vi "KH7008 Control Panel.vi"() -> ()   [LabVIEW 2013]
uses:
  <vilib>/Utility/xml.llb/Write to XML File(string).vi
  <vilib>/Utility/xml.llb/Read From XML File(string).vi
panel:
  in  "Device Number":i32=113885
  in  "Old Settings":T1(array[cluster])=[{"Gain"=1, "Input Coupling"=3, "Shunt Resistor"=1, "Coupling"=1, "Bandwidth Filter"=2}, {"Gain"=1, "Input Coupling"=3, "Shunt Resistor"=1, "Coupling"=1, "Bandwidth Filter"=2}, {"Gain"=1, "Input Coupling"=3, "Shunt Resistor"=1, "Coupling"=1, "Bandwidth Filter"=2}, {"Gain"=1, "Input Coupling"=3, "Shunt Resistor"=1, "Coupling"=1, "Bandwidth Filter"=2}, {"Gain"=1, "Input Coupling"=3, "Shunt Resistor"=1, "Coupling"=1, "Bandwidth Filter"=2}, {"Gain"=1, "Input Coupling"=3, "Shunt Resistor"=1, "Coupling"=1, "Bandwidth Filter"=2}, {"Gain"=1, "Input Coupling"=3, "Shunt Resistor"=1, "Coupling"=1, "Bandwidth Filter"=2}, {"Gain"=1, "Input Coupling"=3, "Shunt Resistor"=1, "Coupling"=1, "Bandwidth Filter"=2}] {"Bandwidth Filter" items=["OFF"=1, "ON"=2]; "Coupling" items=["AC"=1, "DC"=2]; "Shunt Resistor" items=["Open"=1, "50"=2, "500"=3, "5k"=4, "50k"=5]; "Input Coupling" items=["Off"=1, "SE +"=2, "SE -"=3, "Diff"=4]; "Gain" items=["1x"=1, "10x"=2, "100x"=3, "1000x"=4]}
  in  "Load":bool
  in  "Save":bool
  in  "File Identifier (for save)":string
  out "Working":bool
  in  "Refresh":bool
  in  "Settings":T1(array[cluster])=[{"Gain"=1, "Input Coupling"=3, "Shunt Resistor"=1, "Coupling"=1, "Bandwidth Filter"=2}, {"Gain"=1, "Input Coupling"=3, "Shunt Resistor"=1, "Coupling"=1, "Bandwidth Filter"=2}, {"Gain"=1, "Input Coupling"=3, "Shunt Resistor"=1, "Coupling"=1, "Bandwidth Filter"=2}, {"Gain"=1, "Input Coupling"=3, "Shunt Resistor"=1, "Coupling"=1, "Bandwidth Filter"=2}, {"Gain"=1, "Input Coupling"=3, "Shunt Resistor"=1, "Coupling"=1, "Bandwidth Filter"=2}, {"Gain"=1, "Input Coupling"=3, "Shunt Resistor"=1, "Coupling"=1, "Bandwidth Filter"=2}, {"Gain"=1, "Input Coupling"=3, "Shunt Resistor"=1, "Coupling"=1, "Bandwidth Filter"=2}, {"Gain"=1, "Input Coupling"=3, "Shunt Resistor"=1, "Coupling"=1, "Bandwidth Filter"=2}] {"Bandwidth Filter" items=["OFF"=1, "ON"=2]; "Coupling" items=["AC"=1, "DC"=2]; "Shunt Resistor" items=["Open"=1, "50"=2, "500"=3, "5k"=4, "50k"=5]; "Input Coupling" items=["Off"=1, "SE +"=2, "SE -"=3, "Diff"=4]; "Gain" items=["1x"=1, "10x"=2, "100x"=3, "1000x"=4]}
  in  "VISA resource name":refnum<visa-resource-name>="COM3"
  # "Input\nCoupling"
  # "Shunt\nResistor"
  # "Bandwidth\nFilter"
  # "Gain"
  # "Coupling"
  # "CH 1"
  # "CH 2"
  # "CH 3"
  # "CH 4"
  # "CH 5"
  # "CH 6"
  # "CH 7"
  # "CH 8"
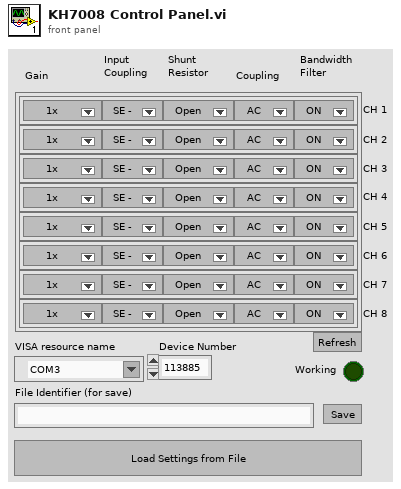
[diagram p1: front panel]
types:
  T1 = cluster{"Gain":u16, "Input Coupling":u16, "Shunt Resistor":u16, "Coupling":u16, "Bandwidth Filter":u16}[]
  T2 = cluster{"Gain":u16, "Input Coupling":u16, "Shunt Resistor":u16, "Coupling":u16, "Bandwidth Filter":u16}
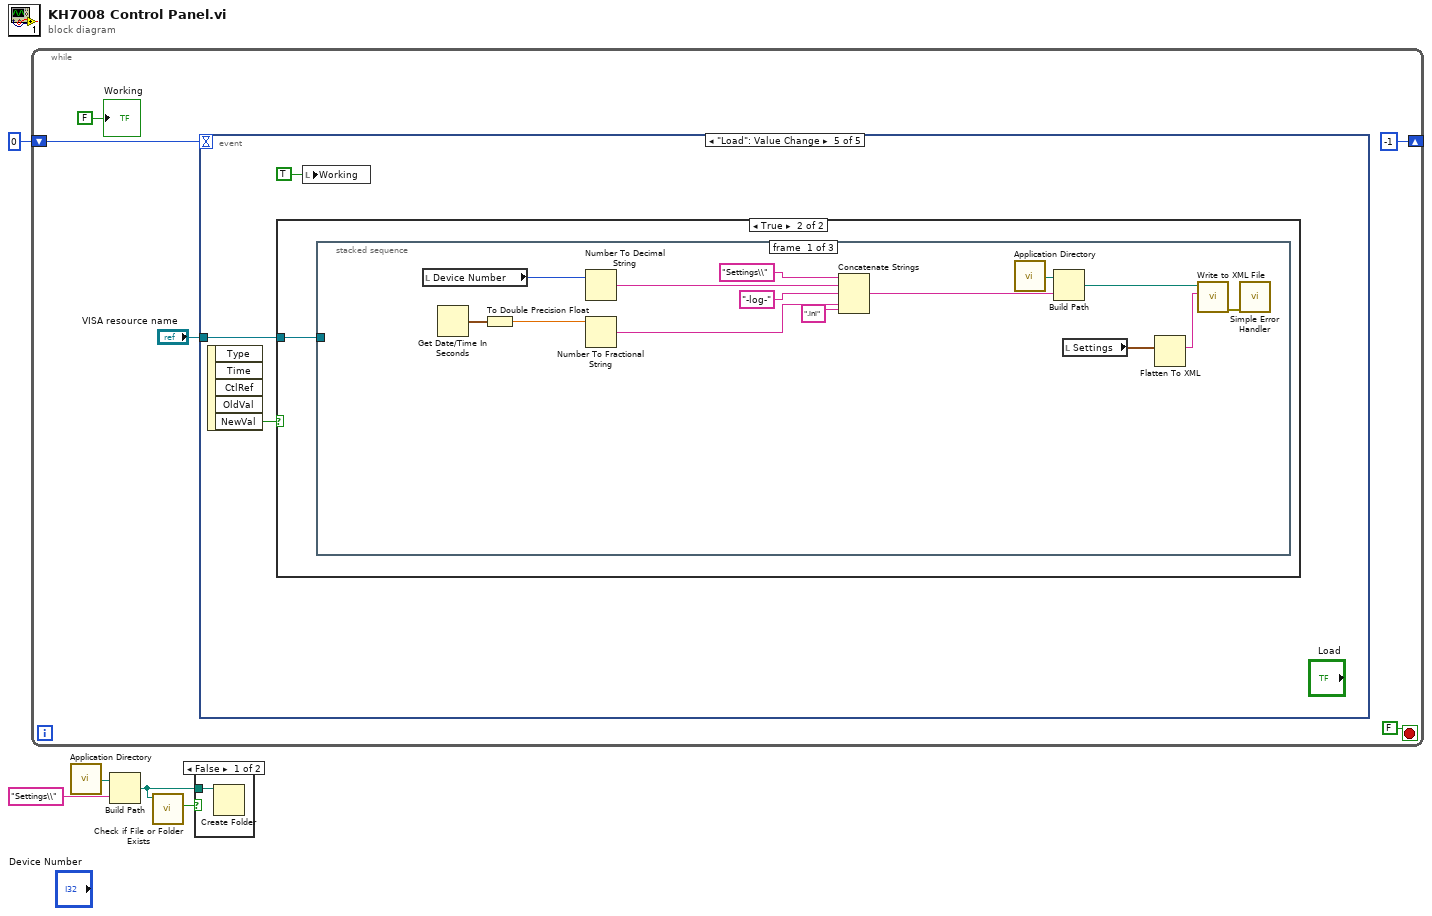
[diagram p0: block diagram]
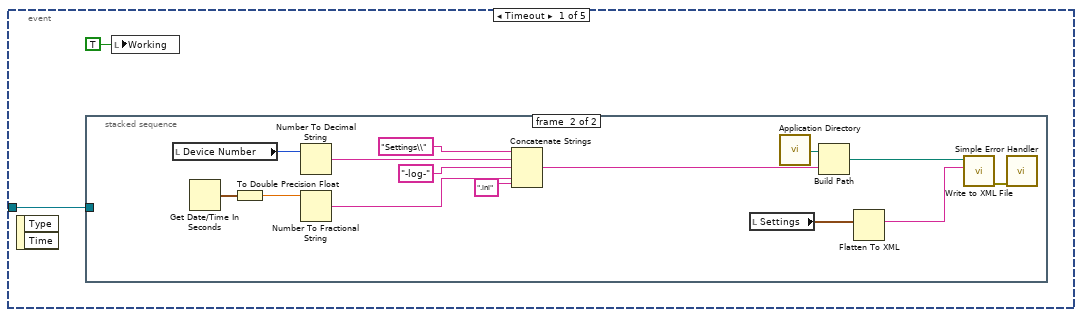
[diagram p3: hidden frame]
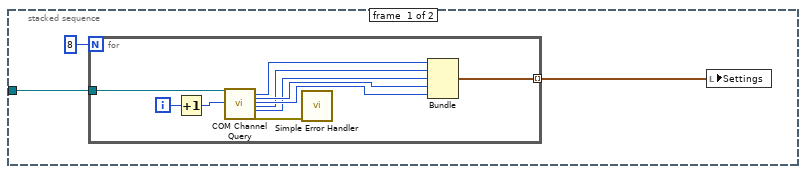
[diagram p4: hidden frame]
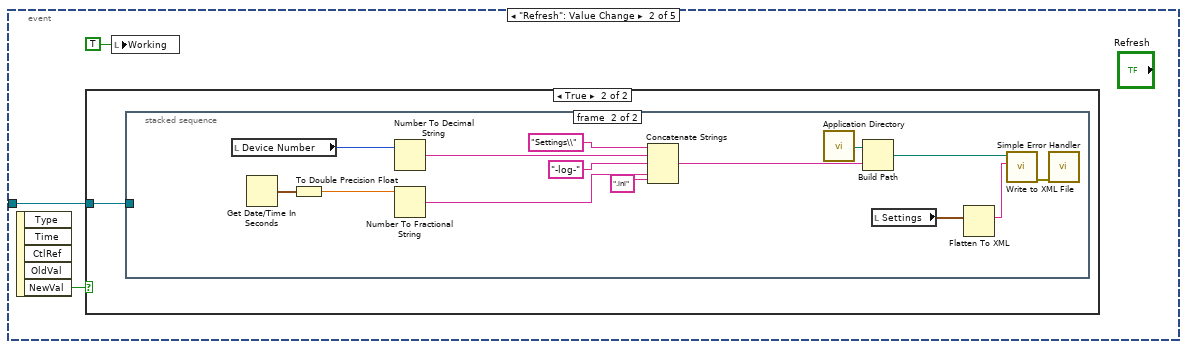
[diagram p5: hidden frame]
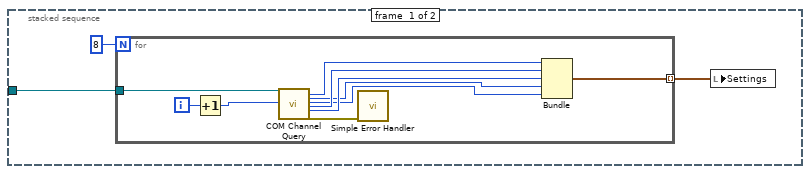
[diagram p7: hidden frame]
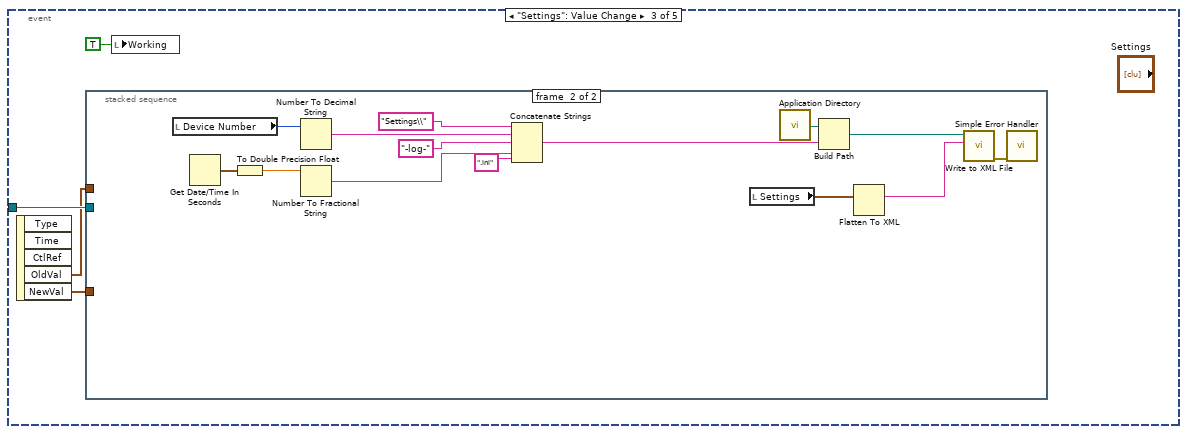
[diagram p8: hidden frame]
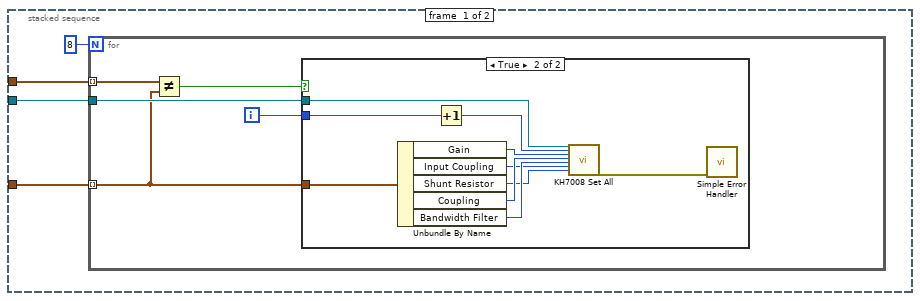
[diagram p9: hidden frame]
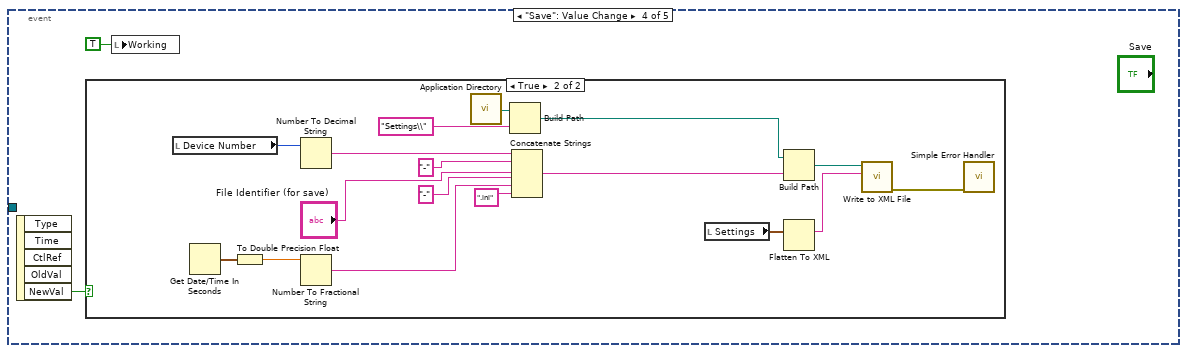
[diagram p11: hidden frame]
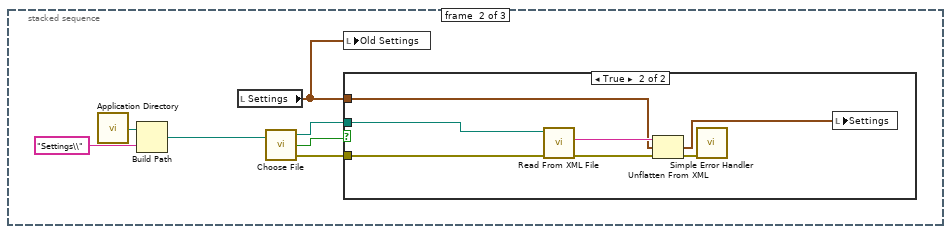
[diagram p14: hidden frame]
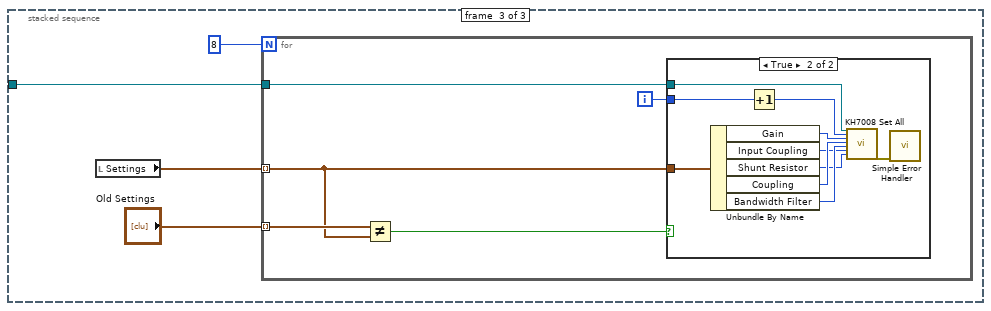
[diagram p16: hidden frame]
diagram:
  n1 = while {
    shift-right: [-1] -> _
    shift-left: 0 -> [w9]
    stop <- FALSE stop-if-true
    n2 = event shown="[4] \"Load\": Value Change" {
      selector: _ -> [_ _ _ _ _]
      dyn-events: _ -> [_ _ _ _ _]
      timeout: w9 -> [_ _ _ _ _]
      tunnel: "VISA resource name" -> [w12 w41 w74 _ w128]
      event Timeout {
        n3 = event-data() -> ()  [unwired: 1 in, 2 out]
        n4 = stacked-sequence {
          tunnel: w12 -> [w15 _]
          frame #0 {
            n5 = for {
              N: 8 -> [_]
              tunnel: w15 -> [w18]
              tunnel: [w16] -> w13 mode=indexing
              i -> [w17]
              n6 = Increment(x=w17) -> (x+1=w19:i32)
              n7 = call <vilib>:"COM Channel Query.vi"("VISA Refnum in"=w18, "Channel"=w19) -> ("Gain"=w21:u16, "Coupling"=w24:u16, "Bandwidth Filter"=w25:u16, "Input Coupling"=w22:u16, "Shunt Resistor"=w23:u16, "error out"=w20:errorcluster)  [unwired: 19 in, 1 out]
              n8 = call <vilib>:"Simple Error Handler.vi"("error in (no error)"=w20) -> ()  [unwired: 4 in, 5 out]
              n9 = Bundle("Gain"=w21, "Input Coupling"=w22, "Shunt Resistor"=w23, "Coupling"=w24, "Bandwidth Filter"=w25) -> (w16:T2)  [unwired: 1 in]
            }
            n10 = local write "Settings"(w13) -> ()
          }
          frame #1 {
            n11 = local read "Device Number"() -> (w28:i32)
            n12 = Get Date/Time In Seconds() -> (seconds since 1Jan1904=w39:timestamp)
            n13 = To Double Precision Float(number=w39) -> (double precision float=w38:dbl)
            n14 = Number To Decimal String(number=w28) -> (decimal integer string=w26:string)  [unwired: 1 in]
            n15 = Number To Fractional String(number=w38) -> (F-format string=w30:string)  [unwired: 3 in]
            n16 = Concatenate Strings("Settings\\", w26, "-log-" ("string"), w30, ".ini" ("string")) -> (w33:string)
            n17 = local read "Settings"() -> (w34:T1)
            n18 = call <vilib>:"Application Directory.vi"() -> ("Application Directory"=w37:path)
            n19 = Build Path(base path=w37, name or relative path=w33) -> (appended path=w32:path)
            n20 = Flatten To XML(anything=w34) -> (xml string=w35:string)
            n21 = call-poly <vilib>:"Write to XML File.vi"("XML Input"=w35, "XML File Path"=w32) -> ("error out"=w36:errorcluster)  [unwired: 7 in, 2 out]
            n22 = call <vilib>:"Simple Error Handler.vi"("error in (no error)"=w36) -> ()  [unwired: 4 in, 5 out]
          }
        }
        n23 = local write "Working"(TRUE ("Working")) -> ()
      }
      event "Refresh": Value Change {
        n24 = event-data() -> ("NewVal"=w42:bool)  [unwired: 1 in, 4 out]
        n25 = case shown="True" w42 {
          tunnel: w41 -> [_ w43]
          frame False {
          }
          frame True {
            n26 = stacked-sequence {
              tunnel: w43 -> [w45 _]
              frame #0 {
                n27 = for {
                  N: 8 -> [_]
                  tunnel: w45 -> [w54]
                  tunnel: [w52] -> w44 mode=indexing
                  i -> [w56]
                  n28 = Increment(x=w56) -> (x+1=w55:i32)
                  n29 = call <vilib>:"COM Channel Query.vi"("VISA Refnum in"=w54, "Channel"=w55) -> ("Gain"=w51:u16, "Coupling"=w48:u16, "Bandwidth Filter"=w47:u16, "Input Coupling"=w50:u16, "Shunt Resistor"=w49:u16, "error out"=w53:errorcluster)  [unwired: 19 in, 1 out]
                  n30 = call <vilib>:"Simple Error Handler.vi"("error in (no error)"=w53) -> ()  [unwired: 4 in, 5 out]
                  n31 = Bundle("Gain"=w51, "Input Coupling"=w50, "Shunt Resistor"=w49, "Coupling"=w48, "Bandwidth Filter"=w47) -> (w52:T2)  [unwired: 1 in]
                }
                n32 = local write "Settings"(w44) -> ()
              }
              frame #1 {
                n33 = local read "Device Number"() -> (w58:i32)
                n34 = Get Date/Time In Seconds() -> (seconds since 1Jan1904=w65:timestamp)
                n35 = To Double Precision Float(number=w65) -> (double precision float=w64:dbl)
                n36 = Number To Decimal String(number=w58) -> (decimal integer string=w57:string)  [unwired: 1 in]
                n37 = Number To Fractional String(number=w64) -> (F-format string=w61:string)  [unwired: 3 in]
                n38 = Concatenate Strings("Settings\\", w57, "-log-" ("string"), w61, ".ini" ("string")) -> (w59:string)
                n39 = call <vilib>:"Application Directory.vi"() -> ("Application Directory"=w69:path)
                n40 = Build Path(base path=w69, name or relative path=w59) -> (appended path=w70:path)
                n41 = local read "Settings"() -> (w66:T1)
                n42 = Flatten To XML(anything=w66) -> (xml string=w67:string)
                n43 = call-poly <vilib>:"Write to XML File.vi"("XML Input"=w67, "XML File Path"=w70) -> ("error out"=w68:errorcluster)  [unwired: 7 in, 2 out]
                n44 = call <vilib>:"Simple Error Handler.vi"("error in (no error)"=w68) -> ()  [unwired: 4 in, 5 out]
              }
            }
          }
        }
        n45 = local write "Working"(TRUE ("Working")) -> ()
      }
      event "Settings": Value Change {
        n46 = event-data() -> ("OldVal"=w71:T1, "NewVal"=w73:T1)  [unwired: 1 in, 3 out]
        n47 = stacked-sequence {
          tunnel: w74 -> [w78 _]
          tunnel: w73 -> [w75 _]
          tunnel: w71 -> [w76 _]
          frame #0 {
            n48 = for {
              N: 8 -> [_]
              tunnel: w78 -> [w83]
              tunnel: w75 -> [w80] mode=indexing
              tunnel: w76 -> [w81] mode=indexing
              i -> [w82]
              n49 = Not Equal?(x=w81, y=w80) -> (x != y?=w79:bool)
              n50 = case shown="True" w79 {
                tunnel: w83 -> [_ w93]
                tunnel: w82 -> [_ w92]
                tunnel: w80 -> [_ w84]
                frame False {
                }
                frame True {
                  n51 = Unbundle By Name(w84) -> ("Gain"=w90:u16, "Input Coupling"=w87:u16, "Shunt Resistor"=w86:u16, "Coupling"=w89:u16, "Bandwidth Filter"=w88:u16)
                  n52 = Increment(x=w92) -> (x+1=w91:i32)
                  n53 = call <vilib>:"KH7008 Set All.vi"("VISA Refnum in"=w93, "Channel"=w91, "Gain"=w90, "Coupling"=w89, "Bandwidth Filter"=w88, "Input Coupling"=w87, "Shunt Resistor"=w86) -> ("error out"=w85:errorcluster)  [unwired: 20 in]
                  n54 = call <vilib>:"Simple Error Handler.vi"("error in (no error)"=w85) -> ()  [unwired: 4 in, 5 out]
                }
              }
            }
          }
          frame #1 {
            n55 = local read "Device Number"() -> (w95:i32)
            n56 = Get Date/Time In Seconds() -> (seconds since 1Jan1904=w102:timestamp)
            n57 = To Double Precision Float(number=w102) -> (double precision float=w101:dbl)
            n58 = Number To Decimal String(number=w95) -> (decimal integer string=w94:string)  [unwired: 1 in]
            n59 = Number To Fractional String(number=w101) -> (F-format string=w98:string)  [unwired: 3 in]
            n60 = Concatenate Strings("Settings\\", w94, "-log-" ("string"), w98, ".ini" ("string")) -> (w96:string)
            n61 = local read "Settings"() -> (w103:T1)
            n62 = call <vilib>:"Application Directory.vi"() -> ("Application Directory"=w106:path)
            n63 = Build Path(base path=w106, name or relative path=w96) -> (appended path=w107:path)
            n64 = Flatten To XML(anything=w103) -> (xml string=w104:string)
            n65 = call-poly <vilib>:"Write to XML File.vi"("XML Input"=w104, "XML File Path"=w107) -> ("error out"=w105:errorcluster)  [unwired: 7 in, 2 out]
            n66 = call <vilib>:"Simple Error Handler.vi"("error in (no error)"=w105) -> ()  [unwired: 4 in, 5 out]
          }
        }
        n67 = local write "Working"(TRUE ("Working")) -> ()
      }
      event "Save": Value Change {
        n68 = event-data() -> ("NewVal"=w108:bool)  [unwired: 1 in, 4 out]
        n69 = case shown="True" w108 {
          frame False {
          }
          frame True {
            n70 = local read "Device Number"() -> (w111:i32)
            n71 = Get Date/Time In Seconds() -> (seconds since 1Jan1904=w123:timestamp)
            n72 = To Double Precision Float(number=w123) -> (double precision float=w119:dbl)
            n73 = Number To Decimal String(number=w111) -> (decimal integer string=w110:string)  [unwired: 1 in]
            n74 = Number To Fractional String(number=w119) -> (F-format string=w122:string)  [unwired: 3 in]
            n75 = call <vilib>:"Application Directory.vi"() -> ("Application Directory"=w118:path)
            n76 = Build Path(base path=w118, name or relative path="Settings\\") -> (appended path=w116:path)
            n77 = Concatenate Strings(w110, "-" ("string"), "File Identifier (for save)", "-" ("string"), w122, ".ini" ("string")) -> (w115:string)
            n78 = local read "Settings"() -> (w126:T1)
            n79 = Build Path(base path=w116, name or relative path=w115) -> (appended path=w114:path)
            n80 = Flatten To XML(anything=w126) -> (xml string=w125:string)
            n81 = call-poly <vilib>:"Write to XML File.vi"("XML Input"=w125, "XML File Path"=w114) -> ("error out"=w124:errorcluster)  [unwired: 7 in, 2 out]
            n82 = call <vilib>:"Simple Error Handler.vi"("error in (no error)"=w124) -> ()  [unwired: 4 in, 5 out]
          }
        }
        n83 = local write "Working"(TRUE ("Working")) -> ()
      }
      event "Load": Value Change {
        n84 = event-data() -> ("NewVal"=w129:bool)  [unwired: 1 in, 4 out]
        n85 = case shown="True" w129 {
          tunnel: w128 -> [_ w130]
          frame False {
          }
          frame True {
            n86 = stacked-sequence {
              tunnel: w130 -> [_ _ w159]
              frame #0 {
                n87 = local read "Device Number"() -> (w132:i32)
                n88 = Get Date/Time In Seconds() -> (seconds since 1Jan1904=w138:timestamp)
                n89 = To Double Precision Float(number=w138) -> (double precision float=w139:dbl)
                n90 = Number To Decimal String(number=w132) -> (decimal integer string=w131:string)  [unwired: 1 in]
                n91 = Number To Fractional String(number=w139) -> (F-format string=w142:string)  [unwired: 3 in]
                n92 = Concatenate Strings("Settings\\", w131, "-log-" ("string"), w142, ".ini" ("string")) -> (w144:string)
                n93 = call <vilib>:"Application Directory.vi"() -> ("Application Directory"=w135:path)
                n94 = Build Path(base path=w135, name or relative path=w144) -> (appended path=w134:path)
                n95 = local read "Settings"() -> (w133:T1)
                n96 = Flatten To XML(anything=w133) -> (xml string=w137:string)
                n97 = call-poly <vilib>:"Write to XML File.vi"("XML Input"=w137, "XML File Path"=w134) -> ("error out"=w136:errorcluster)  [unwired: 7 in, 2 out]
                n98 = call <vilib>:"Simple Error Handler.vi"("error in (no error)"=w136) -> ()  [unwired: 4 in, 5 out]
              }
              frame #1 {
                n99 = call <vilib>:"Application Directory.vi"() -> ("Application Directory"=w151:path)
                n100 = Build Path(base path=w151, name or relative path="Settings\\") -> (appended path=w149:path)
                n101 = local read "Settings"() -> (w145:T1)
                n102 = call <vilib>:"Choose File.vi"("Search Directory"=w149) -> ("Return Path"=w148:path, "Loaded"=w146:bool, "error out"=w147:errorcluster)  [unwired: 1 in]
                n103 = local write "Old Settings"(w145) -> ()
                n104 = case shown="True" w146 {
                  tunnel: w148 -> [_ w158]
                  tunnel: w147 -> [_ w157]
                  tunnel: w145 -> [_ w152]
                  frame False {
                  }
                  frame True {
                    n105 = call-poly <vilib>:"Read From XML File.vi"("error in (no error)"=w157, "XML File Path"=w158) -> ("error out"=w154:errorcluster, "XML Elements"=w156:string)  [unwired: 7 in, 1 out]
                    n106 = Unflatten From XML(xml string=w156, type=w152, error in (no error)=w154) -> (value=w155:T1, error out=w153:errorcluster)
                    n107 = call <vilib>:"Simple Error Handler.vi"("error in (no error)"=w153) -> ()  [unwired: 4 in, 5 out]
                    n108 = local write "Settings"(w155) -> ()
                  }
                }
              }
              frame #2 {
                n109 = local read "Settings"() -> (w160:T1)
                n110 = for {
                  N: 8 -> [_]
                  tunnel: "Old Settings" -> [w166] mode=indexing
                  tunnel: w160 -> [w165] mode=indexing
                  tunnel: w159 -> [w164]
                  i -> [w163]
                  n111 = Not Equal?(x=w166, y=w165) -> (x != y?=w167:bool)
                  n112 = case shown="True" w167 {
                    tunnel: w164 -> [_ w177]
                    tunnel: w165 -> [_ w169]
                    tunnel: w163 -> [_ w168]
                    frame False {
                    }
                    frame True {
                      n113 = Unbundle By Name(w169) -> ("Gain"=w175:u16, "Input Coupling"=w172:u16, "Shunt Resistor"=w171:u16, "Coupling"=w174:u16, "Bandwidth Filter"=w173:u16)
                      n114 = Increment(x=w168) -> (x+1=w176:i32)
                      n115 = call <vilib>:"KH7008 Set All.vi"("VISA Refnum in"=w177, "Channel"=w176, "Gain"=w175, "Coupling"=w174, "Bandwidth Filter"=w173, "Input Coupling"=w172, "Shunt Resistor"=w171) -> ("error out"=w170:errorcluster)  [unwired: 20 in]
                      n116 = call <vilib>:"Simple Error Handler.vi"("error in (no error)"=w170) -> ()  [unwired: 4 in, 5 out]
                    }
                  }
                }
              }
            }
          }
        }
        n117 = local write "Working"(TRUE ("Working")) -> ()
      }
    }
    "Working" <- FALSE ("Working")
  }
  n118 = call <vilib>:"Application Directory.vi"() -> ("Application Directory"=w3:path)
  n119 = Build Path(base path=w3, name or relative path="Settings\\") -> (appended path=w2:path)
  n120 = call <vilib>:"Check if File or Folder Exists.vi"("path"=w2) -> ("file or folder exists?"=w1:bool)  [unwired: 8 in, 2 out]
  n121 = case shown="False" w1 {
    tunnel: w2 -> [w178 _]
    frame False {
      n122 = Create Folder(path (use dialog)=w178) -> ()  [unwired: 2 in, 3 out]
    }
    frame True {
    }
  }
